vi "SeCrTS-DD NS Data.vi"(7 "NOT DIS Out":T1, 8 "error in":errorcluster, 9 "AI_V_Data P\nAI_C_Data P\nAO_Data P\nDO_Data P\nACC_Data P\nTC Data P\nDrive_A_C \nDrive_A_D\nAI_C_Data S\nDO_Data S\nAI_V_Rms_P":refnum<queue>[](array[refnum]), 10 "data out":string, 11 "DI P\nDI S":refnum<queue>[](array[refnum])) -> (0 "error out":errorcluster)   [LabVIEW 2022 SP3]
uses:
  Control/SeCrTS-Notifier Ref.ctl
panel:
  out "overflow? 10":bool
  out "overflow? 9":bool
  out "overflow? 8":bool
  out "overflow? 7":bool
  out "overflow? 6":bool
  out "overflow? 5":bool
  out "overflow? 4":bool
  out "overflow? 3":bool
  out "overflow? 2":bool
  out "overflow?":bool
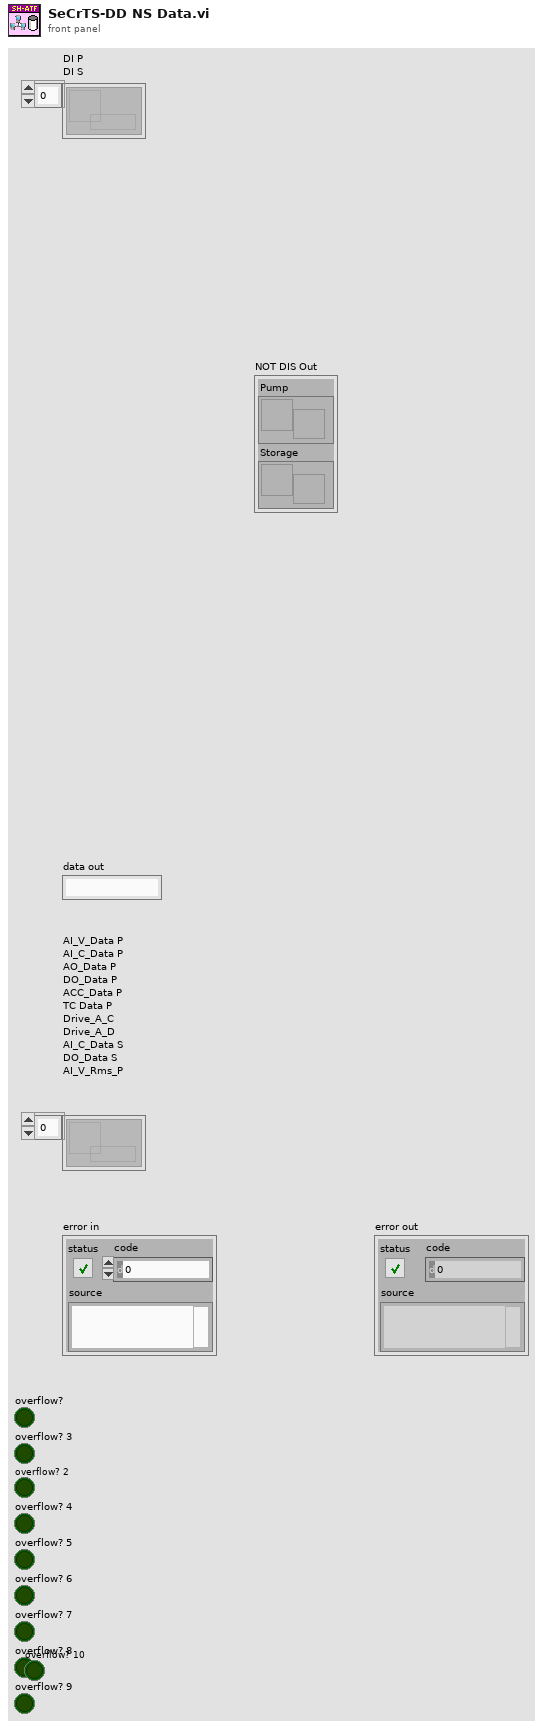
[diagram p1: front panel]
types:
  T1 = typedef "SeCrTS-Notifier Ref.ctl" = cluster{"Pump":refnum<notifier>, "Storage":refnum<notifier>}
  T2 = cluster{"AI_V_Data":waveform(dbl)[][], "AI_C_Data":waveform(dbl)[][], "AO_Data":waveform(dbl)[][], "DO_Data":waveform(dbl)[][], "DI_Data":digitalwaveform[][], "ACC_Data":waveform(dbl)[][], "TC Data":waveform(dbl)[][], "Drive_A_C":waveform(dbl)[][], "Drive_A_D":waveform(dbl)[][], "AI_V Rms":waveform(dbl)[][]}
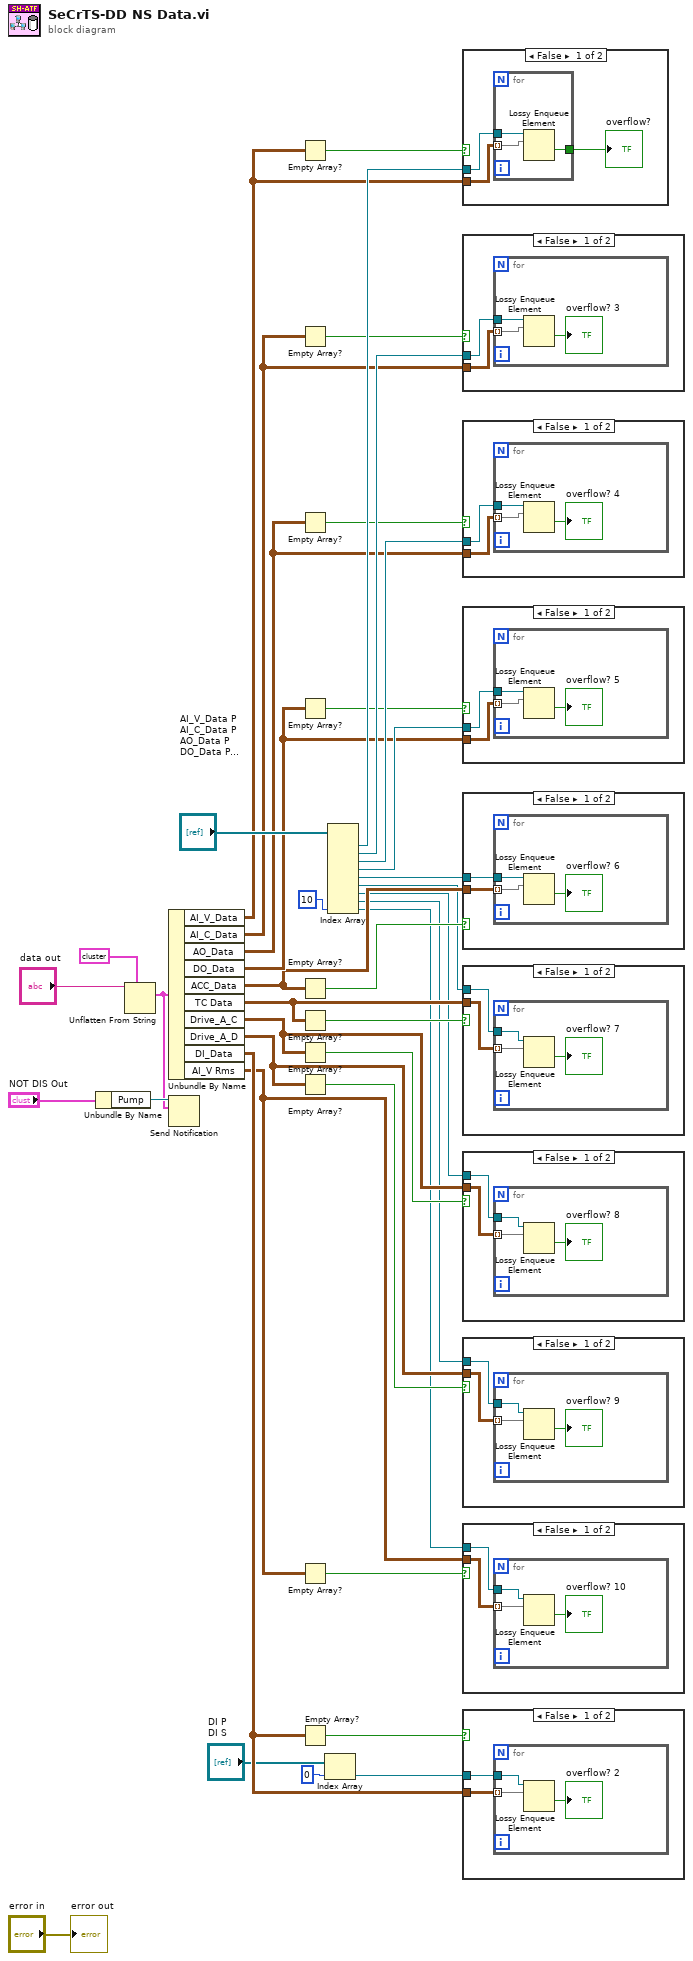
[diagram p0: block diagram]
diagram:
  n1 = Unbundle By Name("NOT DIS Out") -> ("Pump"=w3:refnum<notifier>)
  n2 = Unflatten From String(type=T2 data[101840B] ("data out 2"), binary string="data out") -> (value=w2:T2)  [unwired: 3 in, 2 out]
  n3 = Unbundle By Name(w2) -> ("AI_V_Data"=w32:waveform(dbl)[][], "AI_C_Data"=w34:waveform(dbl)[][], "AO_Data"=w29:waveform(dbl)[][], "DO_Data"=w26:waveform(dbl)[][], "ACC_Data"=w24:waveform(dbl)[][], "TC Data"=w21:waveform(dbl)[][], "Drive_A_C"=w18:waveform(dbl)[][], "Drive_A_D"=w15:waveform(dbl)[][], "DI_Data"=w36:digitalwaveform[][], "AI_V Rms"=w6:waveform(dbl)[][])
  n4 = Send Notification(notification=w2, notifier=w3) -> ()  [unwired: 1 in, 2 out]
  n5 = Empty Array?(array=w32) -> (empty?=w33:bool)
  n6 = Empty Array?(array=w34) -> (empty?=w35:bool)
  n7 = Empty Array?(array=w29) -> (empty?=w31:bool)
  n8 = Empty Array?(array=w26) -> (empty?=w28:bool)
  n9 = Empty Array?(array=w24) -> (empty?=w23:bool)
  n10 = Empty Array?(array=w21) -> (empty?=w20:bool)
  n11 = Empty Array?(array=w18) -> (empty?=w17:bool)
  n12 = Empty Array?(array=w15) -> (empty?=w14:bool)
  n13 = Empty Array?(array=w6) -> (empty?=w7:bool)
  n14 = Empty Array?(array=w36) -> (empty?=w37:bool)
  n15 = Index Array(array="DI P\nDI S", index=0) -> (element=w12:refnum<queue>)
  n16 = Index Array(array="AI_V_Data P\nAI_C_Data P\nAO_Data P\nDO_Data P\nACC_Data P\nTC Data P\nDrive_A_C \nDrive_A_D\nAI_C_Data S\nDO_Data S\nAI_V_Rms_P", index #9=10 ("index")) -> (element #1=w39:refnum<queue>, element #2=w40:refnum<queue>, element #3=w30:refnum<queue>, element #4=w27:refnum<queue>, element #5=w25:refnum<queue>, element #6=w22:refnum<queue>, element #7=w19:refnum<queue>, element #8=w16:refnum<queue>, element #9=w5:refnum<queue>)  [unwired: 8 in]
  n17 = case shown="False" w33 {
    tunnel: w32 -> [w43 _]
    tunnel: w39 -> [w42 _]
    frame False {
      n18 = for {
        tunnel: w43 -> [w44] mode=indexing
        tunnel: w42 -> [w46]
        tunnel: [w45] -> w41
        n19 = Lossy Enqueue Element(queue=w46, element=w44) -> (overflow?=w45:bool)  [unwired: 1 in, 3 out]
      }
      "overflow?" <- w41
    }
    frame True {
    }
  }
  n20 = case shown="False" w35 {
    tunnel: w34 -> [w48 _]
    tunnel: w40 -> [w47 _]
    frame False {
      n21 = for {
        tunnel: w48 -> [w49] mode=indexing
        tunnel: w47 -> [w51]
        n22 = Lossy Enqueue Element(queue=w51, element=w49) -> (overflow?=→"overflow? 3":bool)  [unwired: 1 in, 3 out]
      }
    }
    frame True {
    }
  }
  n23 = case shown="False" w31 {
    tunnel: w29 -> [w53 _]
    tunnel: w30 -> [w52 _]
    frame False {
      n24 = for {
        tunnel: w53 -> [w56] mode=indexing
        tunnel: w52 -> [w55]
        n25 = Lossy Enqueue Element(queue=w55, element=w56) -> (overflow?=→"overflow? 4":bool)  [unwired: 1 in, 3 out]
      }
    }
    frame True {
    }
  }
  n26 = case shown="False" w28 {
    tunnel: w26 -> [w58 _]
    tunnel: w27 -> [w57 _]
    frame False {
      n27 = for {
        tunnel: w58 -> [w59] mode=indexing
        tunnel: w57 -> [w61]
        n28 = Lossy Enqueue Element(queue=w61, element=w59) -> (overflow?=→"overflow? 5":bool)  [unwired: 1 in, 3 out]
      }
    }
    frame True {
    }
  }
  n29 = case shown="False" w23 {
    tunnel: w24 -> [w63 _]
    tunnel: w25 -> [w62 _]
    frame False {
      n30 = for {
        tunnel: w63 -> [w64] mode=indexing
        tunnel: w62 -> [w66]
        n31 = Lossy Enqueue Element(queue=w66, element=w64) -> (overflow?=→"overflow? 6":bool)  [unwired: 1 in, 3 out]
      }
    }
    frame True {
    }
  }
  n32 = case shown="False" w20 {
    tunnel: w21 -> [w68 _]
    tunnel: w22 -> [w67 _]
    frame False {
      n33 = for {
        tunnel: w68 -> [w69] mode=indexing
        tunnel: w67 -> [w71]
        n34 = Lossy Enqueue Element(queue=w71, element=w69) -> (overflow?=→"overflow? 7":bool)  [unwired: 1 in, 3 out]
      }
    }
    frame True {
    }
  }
  n35 = case shown="False" w17 {
    tunnel: w18 -> [w73 _]
    tunnel: w19 -> [w72 _]
    frame False {
      n36 = for {
        tunnel: w73 -> [w74] mode=indexing
        tunnel: w72 -> [w76]
        n37 = Lossy Enqueue Element(queue=w76, element=w74) -> (overflow?=→"overflow? 8":bool)  [unwired: 1 in, 3 out]
      }
    }
    frame True {
    }
  }
  n38 = case shown="False" w14 {
    tunnel: w15 -> [w78 _]
    tunnel: w16 -> [w77 _]
    frame False {
      n39 = for {
        tunnel: w78 -> [w79] mode=indexing
        tunnel: w77 -> [w81]
        n40 = Lossy Enqueue Element(queue=w81, element=w79) -> (overflow?=→"overflow? 9":bool)  [unwired: 1 in, 3 out]
      }
    }
    frame True {
    }
  }
  n41 = case shown="False" w7 {
    tunnel: w6 -> [w83 _]
    tunnel: w5 -> [w82 _]
    frame False {
      n42 = for {
        tunnel: w83 -> [w84] mode=indexing
        tunnel: w82 -> [w86]
        n43 = Lossy Enqueue Element(queue=w86, element=w84) -> (overflow?=→"overflow? 10":bool)  [unwired: 1 in, 3 out]
      }
    }
    frame True {
    }
  }
  n44 = case shown="False" w37 {
    tunnel: w36 -> [w88 _]
    tunnel: w12 -> [w87 _]
    frame False {
      n45 = for {
        tunnel: w88 -> [w89] mode=indexing
        tunnel: w87 -> [w91]
        n46 = Lossy Enqueue Element(queue=w91, element=w89) -> (overflow?=→"overflow? 2":bool)  [unwired: 1 in, 3 out]
      }
    }
    frame True {
    }
  }
  "error out" <- "error in"
